vi "Close Reference (Simulate).vi"(8 "error in (no error)":errorcluster, 11 "Instrument Refnum in":refnum<visa-resource-name>) -> (0 "error out":errorcluster)   [LabVIEW 2012]
doc: "Simulates closing a hardware reference"
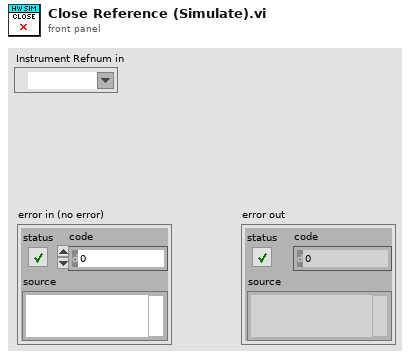
[diagram p1: front panel]
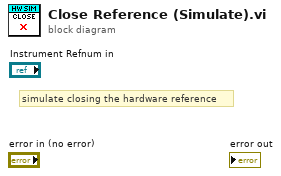
[diagram p0: block diagram]
diagram:
  # "simulate closing the hardware reference"
